vi "WSVCAP SHL Host TL RFFE Configure.vi"(7 "RFFE Slave Address":u8=144 caption="Slave Address" format="0x%02x", 9 "Clock Rate (Hz)":dbl=50000.0, 11 "error in":errorcluster, 13 "Log (T)":bool=TRUE, 14 "FPGA":T1) -> (6 "Actual Rate (Hz)":dbl, 15 "error out":errorcluster)   [LabVIEW 2012]
uses:
  Type Defs/WSVCAP SHL I2C FPGA Enum.ctl
  Type Defs/WSVCAP SHL Function Enum.ctl
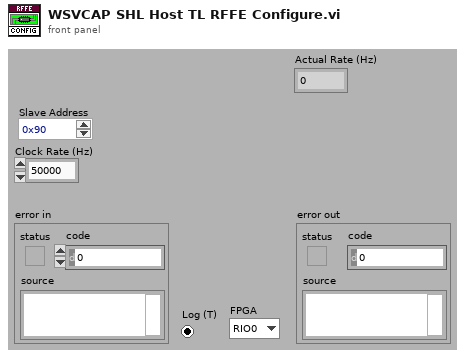
[diagram p1: front panel]
types:
  T1 = typedef "WSVCAP SHL I2C FPGA Enum.ctl" = enum16{"RIO0", "RIO1"}
  T2 = typedef "WSVCAP SHL Function Enum.ctl" = enum16{"Initialize", "Configure I2C", "Configure RFFE", "Write I2C", "Read I2C", "Write RFFE", "Read RFFE", "Start RFFE Cycle", "Stop RFFE Cycle", "Get Status", "Close"}
  T3 = typedef "WSVCAP SHL Core System Cluster.ctl" = cluster{"Settings":T4, "FPGA Resource":tag, "Online":bool, "I2C Wait Ticks":u32, "SPI Wait Ticks":u32, "RFFE Wait Ticks":u32, "FPGA VI Reference (FPGA Mode)":T5, "FPGA VI Reference (Sim Mode)":refnum<vi>}
  T4 = typedef "WSVCAP SHL I2C Settings Cluster.ctl" = cluster{"I2C Slave Address":u8, "I2C Clock Rate (Hz)":dbl, "SPI Clock Rate (Hz)":dbl, "RFFE Slave Address":u8, "RFFE Clock Rate (Hz)":dbl, "Simulate FPGA":bool, "C1 Cap DAC Default":u8, "C2 Cap DAC Default":u8, "C3 Cap DAC Default":u8}
  T5 = typedef "WSVCAP SHL FPGA VI Reference.ctl" = refnum<k20>
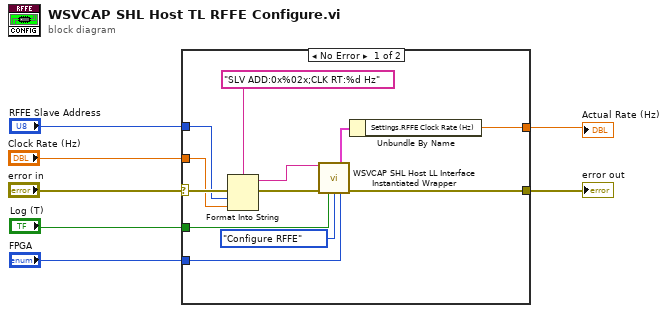
[diagram p0: block diagram]
diagram:
  n1 = case shown="No Error" "error in" {
    selector: "error in" -> [w15 w20]
    tunnel: [w19 w20] -> w7
    tunnel: [w17 _] -> w6
    tunnel: "Clock Rate (Hz)" -> [w13 _]
    tunnel: "Log (T)" -> [w11 _]
    tunnel: "RFFE Slave Address" -> [w9 _]
    tunnel: "FPGA" -> [w8 _]
    frame No Error {
      n2 = Format Into String(format string="SLV ADD:0x%02x;CLK RT:%d Hz", error in=w15, w9, w13) -> (resulting string=w12:string, error out=w14:errorcluster)  [unwired: 1 in]
      n3 = call "WSVCAP SHL Host LL Interface Instantiated Wrapper.vi"("Message In"=w12, "error in"=w14, "Log (T)"=w11, "Function"=WSVCAP_SHL_Function_Enum."Configure RFFE", "FPGA"=w8) -> ("System"=w18:T3, "error out"=w19:errorcluster)  [unwired: 8 in, 1 out]
      n4 = Unbundle By Name(w18) -> ("Settings.RFFE Clock Rate (Hz)"=w17:dbl)
    }
    frame Error {
    }
  }
  "Actual Rate (Hz)" <- w6
  "error out" <- w7
